vi "Graph handler (SubVI).vi"(0 "Data in":dbl[][](array[numeric]), 5 "Graph indices in":dbl[](array[numeric]), 11 "Clear graph Array":bool[](array[boolean])) -> (3 "Graph indices out":dbl[](array[numeric]), 4 "R(T) Graph":cluster{dbl[], dbl[]}(graph), 6 "R(H) Graph":cluster{dbl[], dbl[]}(graph), 8 "R(t) Graph":cluster{dbl[], dbl[]}(graph), 10 "T(t) Graph 3":cluster{dbl[], dbl[]}(graph), 15 "H(t) Graph 4":cluster{dbl[], dbl[]}(graph))   [LabVIEW 2017, in "Fridge Software v2.1.lvlib"]
uses:
  Fridge Software v2.1.lvlib
panel:
  # "R(T)\nR(H)\nR(t)\nT(t)\nH(t)"
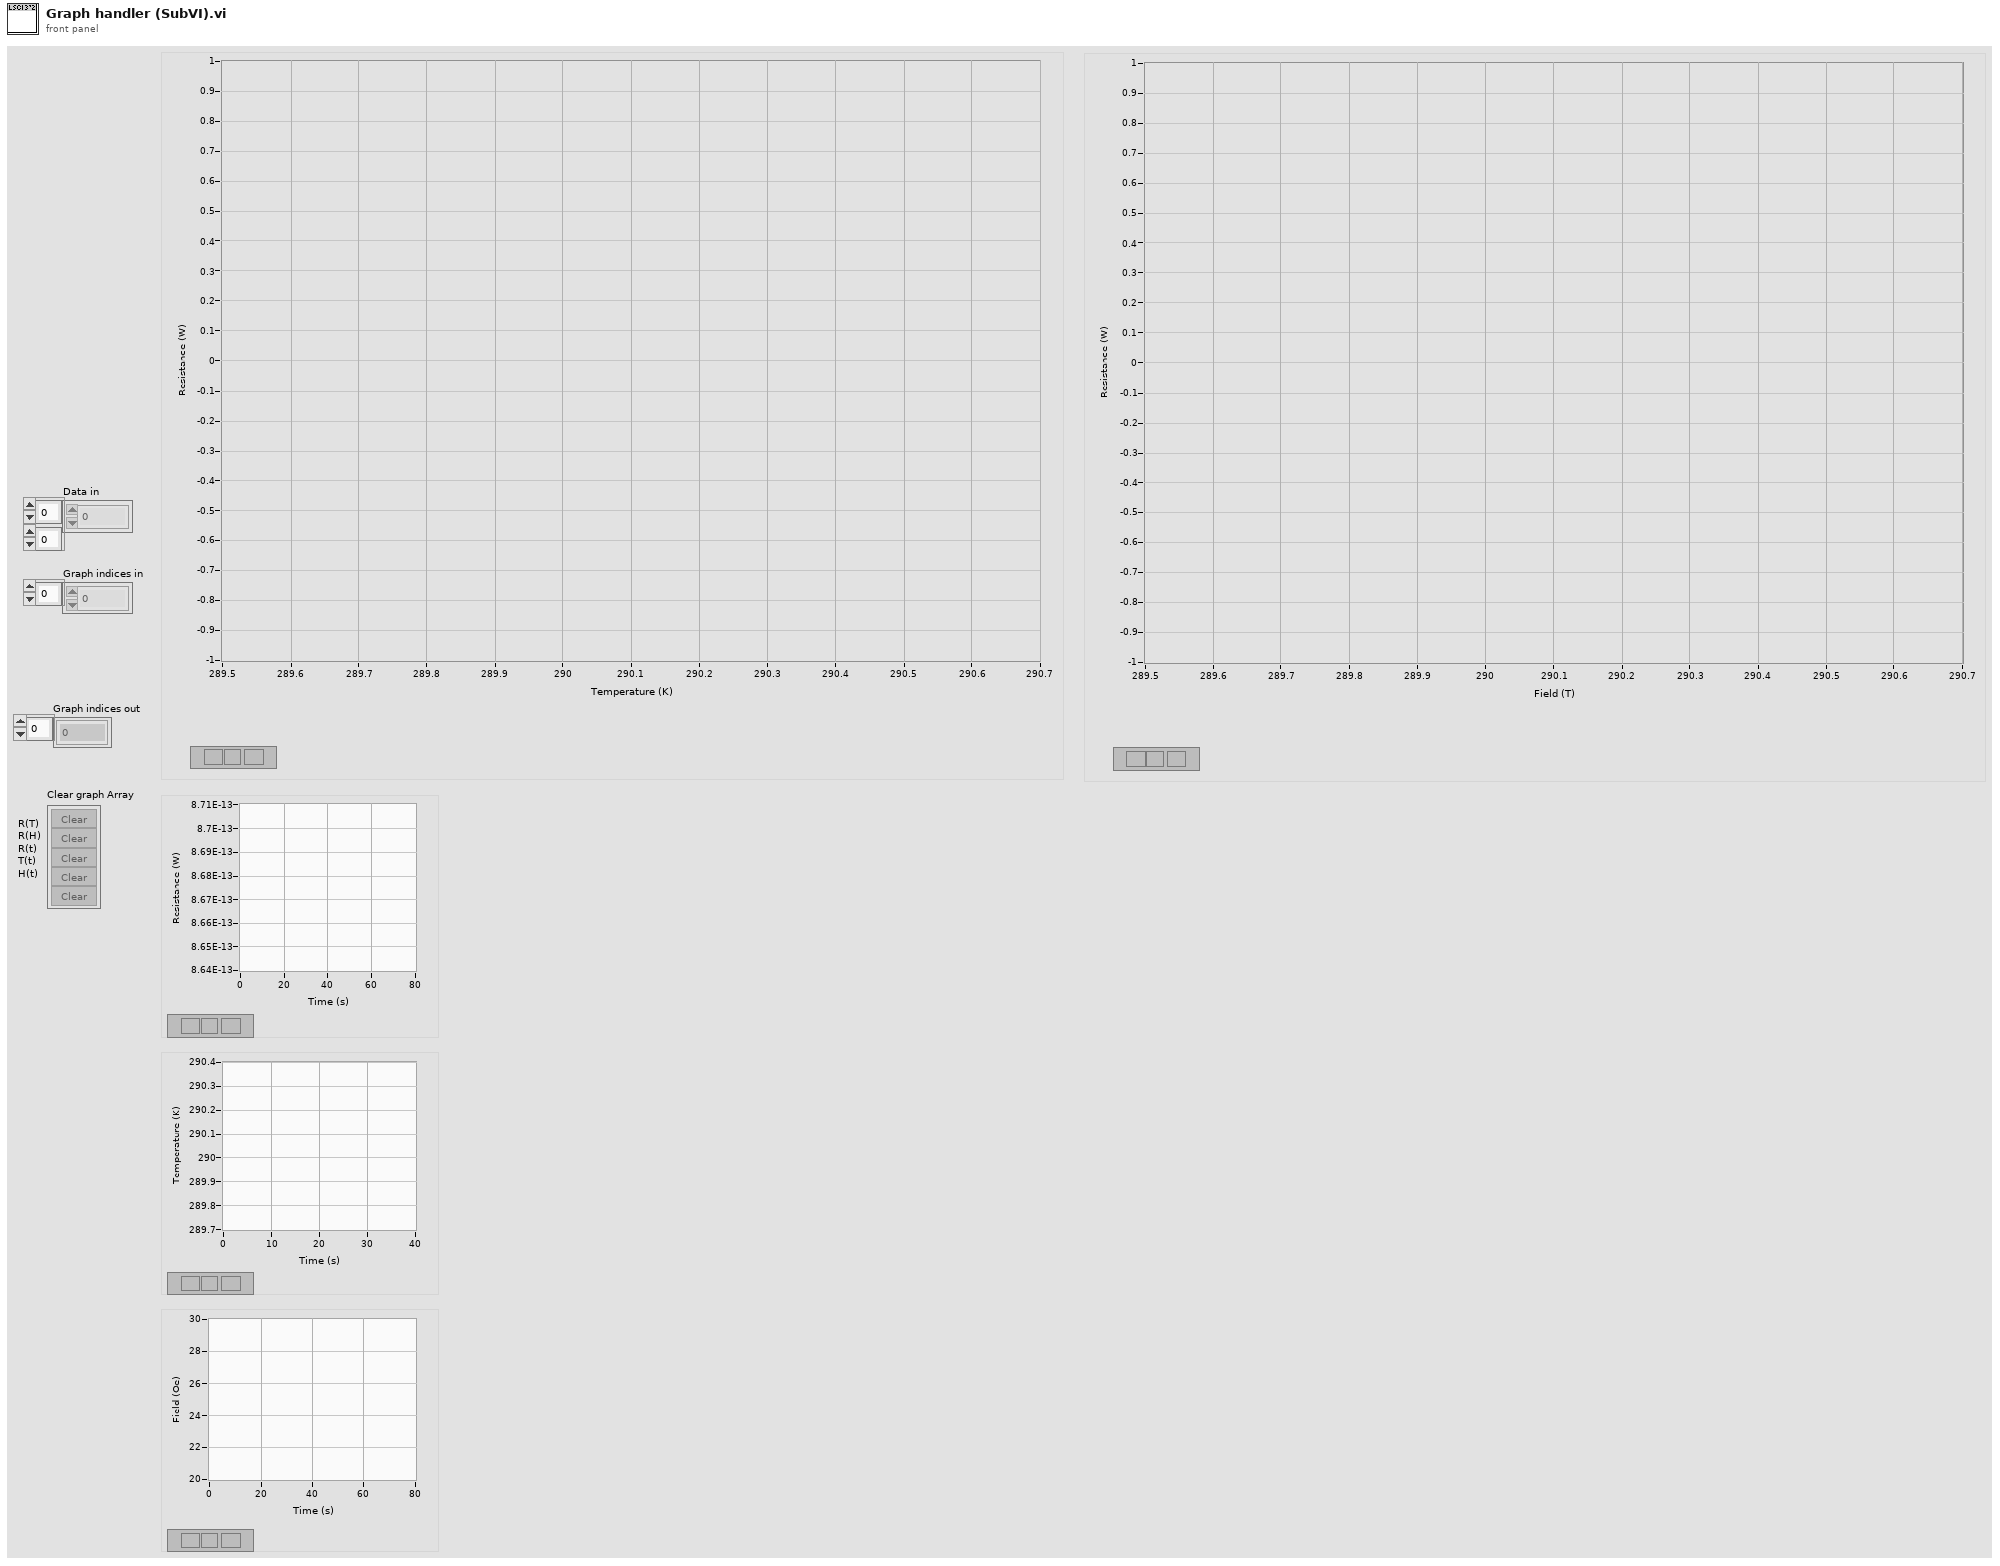
[diagram p1: front panel]
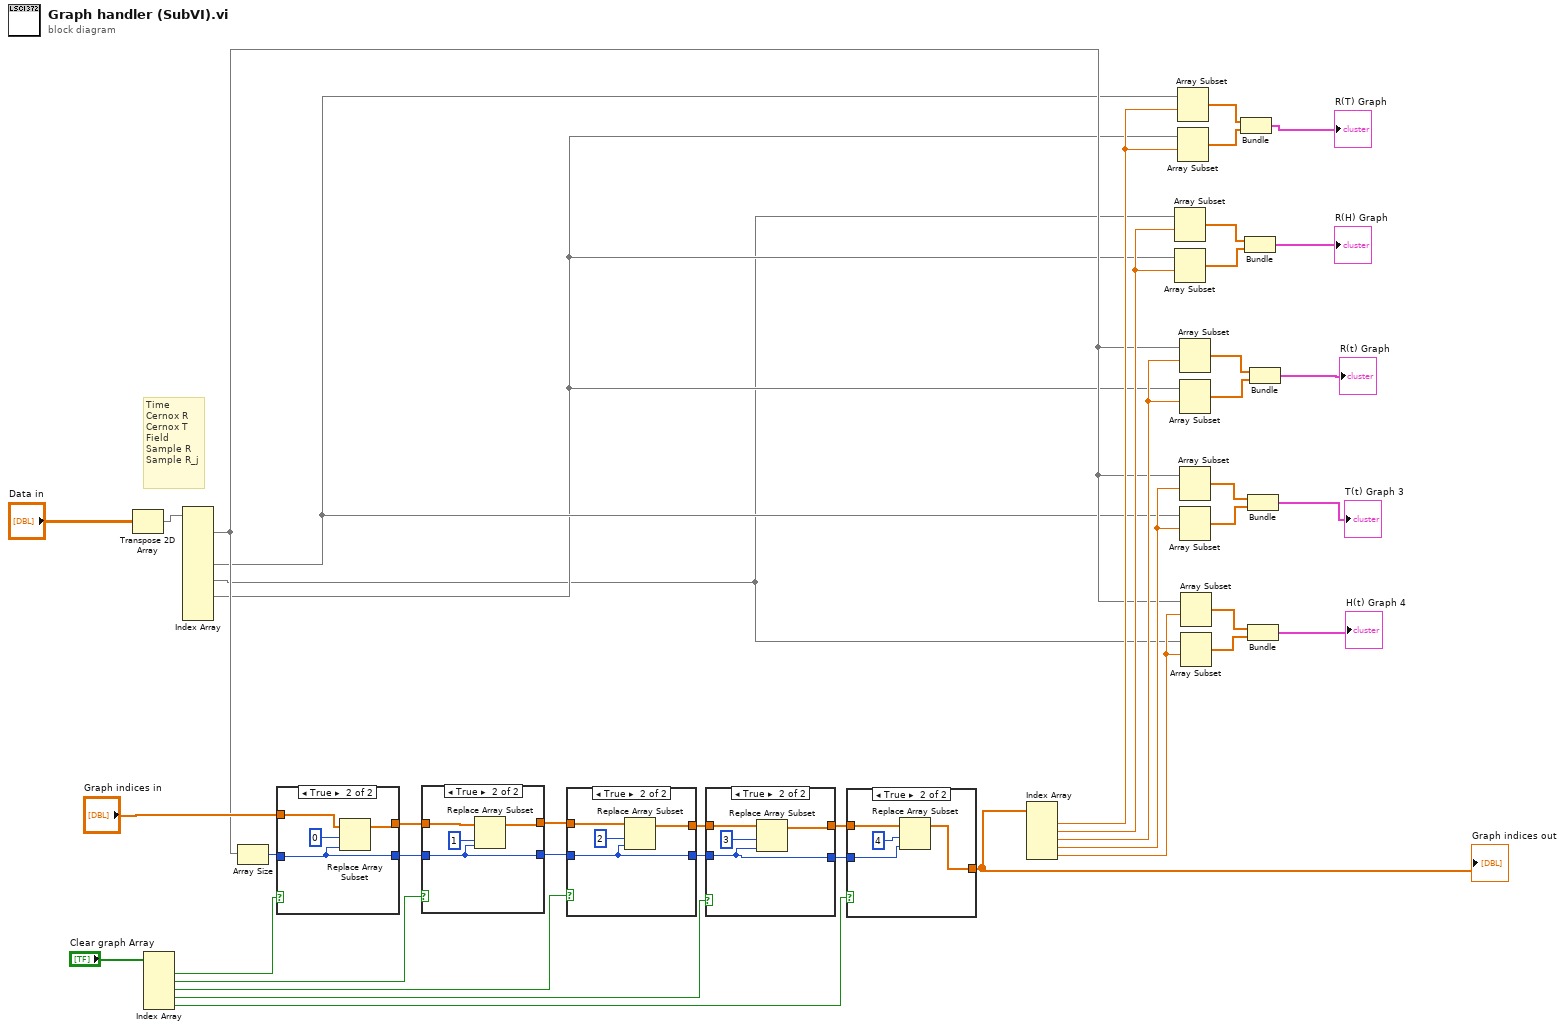
[diagram p0: block diagram]
diagram:
  # "Time\nCernox R\nCernox T\nField\nSample R\nSample R_j"
  n1 = Transpose 2D Array(2D array="Data in") -> (transposed array=w26:dbl[][])
  n2 = Index Array(array="Clear graph Array") -> (element #1=w7:bool, element #2=w6:bool, element #3=w5:bool, element #4=w4:bool, element #5=w3:bool)  [unwired: 5 in]
  n3 = Index Array(array=w26) -> (element #1=w15:dbl[], element #3=w14:dbl[], element #4=w1:dbl[], element #5=w2:dbl[])  [unwired: 12 in, 2 out]
  n4 = Array Size(array=w15) -> (size(s)=w30:i32)
  n5 = case shown="True" w7 {
    tunnel: w30 -> [w44 w46]
    tunnel: "Graph indices in" -> [w45 w49]
    tunnel: [w45 w47] -> w24
    tunnel: [w44 w46] -> w25
    frame False {
    }
    frame True {
      n6 = Replace Array Subset(array=w49, new element=w46, index=0) -> (w47:dbl[])
    }
  }
  n7 = case shown="True" w6 {
    tunnel: w25 -> [w51 w53]
    tunnel: [w50 w54] -> w23
    tunnel: [w51 w53] -> w22
    tunnel: w24 -> [w50 w52]
    frame False {
    }
    frame True {
      n8 = Replace Array Subset(array=w52, new element=w53, index=1) -> (w54:dbl[])
    }
  }
  n9 = case shown="True" w5 {
    tunnel: w23 -> [w57 w58]
    tunnel: [w57 w59] -> w33
    tunnel: w22 -> [w56 w60]
    tunnel: [w56 w60] -> w36
    frame False {
    }
    frame True {
      n10 = Replace Array Subset(array=w58, new element=w60, index=2) -> (w59:dbl[])
    }
  }
  n11 = case shown="True" w4 {
    tunnel: w33 -> [w63 w64]
    tunnel: [w63 w65] -> w34
    tunnel: w36 -> [w62 w67]
    tunnel: [w62 w67] -> w37
    frame False {
    }
    frame True {
      n12 = Replace Array Subset(array=w64, new element=w67, index=3) -> (w65:dbl[])
    }
  }
  n13 = case shown="True" w3 {
    tunnel: w34 -> [w68 w69]
    tunnel: [w68 w70] -> w35
    tunnel: w37 -> [_ w72]
    frame False {
    }
    frame True {
      n14 = Replace Array Subset(array=w69, new element=w72, index=4) -> (w70:dbl[])
    }
  }
  "Graph indices out" <- w35
  n15 = Index Array(array=w35) -> (element #1=w32:dbl, element #2=w16:dbl, element #3=w19:dbl, element #4=w20:dbl, element #5=w21:dbl)  [unwired: 5 in]
  n16 = Array Subset(array=w1, index=w16) -> (w17:dbl[])  [unwired: 1 in]
  n17 = Array Subset(array=w2, index=w16) -> (w18:dbl[])  [unwired: 1 in]
  n18 = Array Subset(array=w14, index=w32) -> (w28:dbl[])  [unwired: 1 in]
  n19 = Array Subset(array=w2, index=w32) -> (w29:dbl[])  [unwired: 1 in]
  n20 = Array Subset(array=w15, index=w19) -> (w40:dbl[])  [unwired: 1 in]
  n21 = Array Subset(array=w2, index=w19) -> (w41:dbl[])  [unwired: 1 in]
  n22 = Array Subset(array=w15, index=w20) -> (w38:dbl[])  [unwired: 1 in]
  n23 = Array Subset(array=w14, index=w20) -> (w39:dbl[])  [unwired: 1 in]
  n24 = Array Subset(array=w15, index=w21) -> (w42:dbl[])  [unwired: 1 in]
  n25 = Array Subset(array=w1, index=w21) -> (w43:dbl[])  [unwired: 1 in]
  n26 = Bundle(w28, w29) -> (→"R(T) Graph":cluster{dbl[], dbl[]})  [unwired: 1 in]
  n27 = Bundle(w17, w18) -> (→"R(H) Graph":cluster{dbl[], dbl[]})  [unwired: 1 in]
  n28 = Bundle(w38, w39) -> (→"T(t) Graph 3":cluster{dbl[], dbl[]})  [unwired: 1 in]
  n29 = Bundle(w42, w43) -> (→"H(t) Graph 4":cluster{dbl[], dbl[]})  [unwired: 1 in]
  n30 = Bundle(w40, w41) -> (→"R(t) Graph":cluster{dbl[], dbl[]})  [unwired: 1 in]
